vi "Destroy Lookup.vi"(8 "error in (no error)":errorcluster, 11 "Lookup Service in":refnum<data-value>) -> (0 "error out":errorcluster)   [LabVIEW 2014, in "LVCOOOP.lvlib" / "Lookup API.lvlib" / "Lookup Service.lvclass"]
doc: "Destroy a Lookup"
uses:
  Lookup Service.lvclass
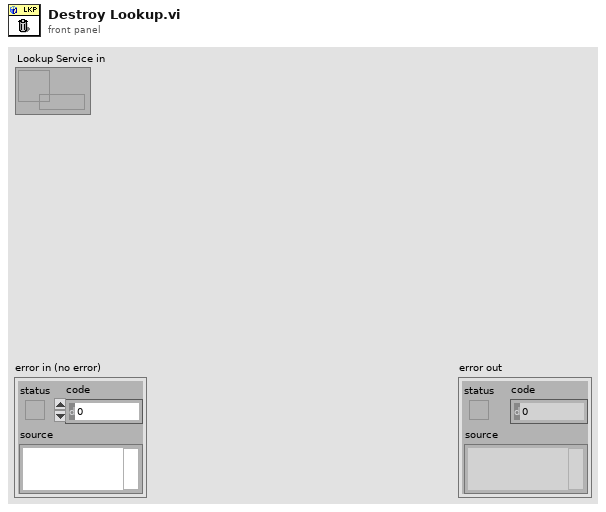
[diagram p1: front panel]
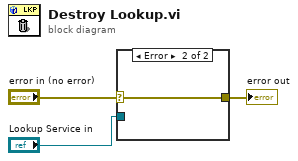
[diagram p0: block diagram]
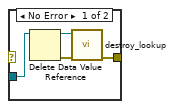
[diagram p2: hidden frame]
diagram:
  n1 = case shown="Error" "error in (no error)" {
    selector: "error in (no error)" -> [_ w8]
    tunnel: "Lookup Service in" -> [w7 _]
    tunnel: [w4 w8] -> w2
    frame No Error {
      n2 = Delete Data Value Reference(data value reference=w7) -> (data value=w6:refnum<class "Lookup Service.lvclass">, error out=w5:errorcluster)  [unwired: 1 in]
      n3 = call-dynamic "destroy_lookup.vi"("error in (no error)"=w5, "Lookup Service in"=w6) -> ("error out"=w4:errorcluster)  [unwired: 9 in]
    }
    frame Error {
    }
  }
  "error out" <- w2
